vi "CRYGraph Property Window Table.vi"(8 "Tab Name":string, 9 "Graph VI Ref":refnum<vi>) -> ()   [LabVIEW 2013]
uses:
  Control/CRYTable Property.ctl
panel:
  in  "Redraw":bool
  in  "Draw":bool
  in  "Table Property":T1 {"Precision" items=["Digits of precision", "Significant digits"]}
  in  "OK":bool
  in  "List Tab":enum32{"Title", "Format"}(tab) caption="Table Tab"
  in  "Title Name":string caption="标题名字"
  in  "Show vertical scroll bar":bool caption="显示垂直滚动条"
  in  "Show horizontal scroll bar":bool caption="显示水平滚动条"
  in  "Row Header Width":u16
  in  "Column Width":u16
  in  "Hide Traling Zeros":bool caption="隐藏尾随零"
  in  "PrecisionType":u16(ring) caption="Precision" items=["精度位数", "有效数字"]
  in  "Digits":u16
  in  "Notation":u16(slide)
  in  "Display Units":bool caption="显示单位"
  in  "Transpose":bool
  in  "Reset All Columns":bool
  out "Number Format":bool caption="数字格式"
  out "Options":bool caption="表选项"
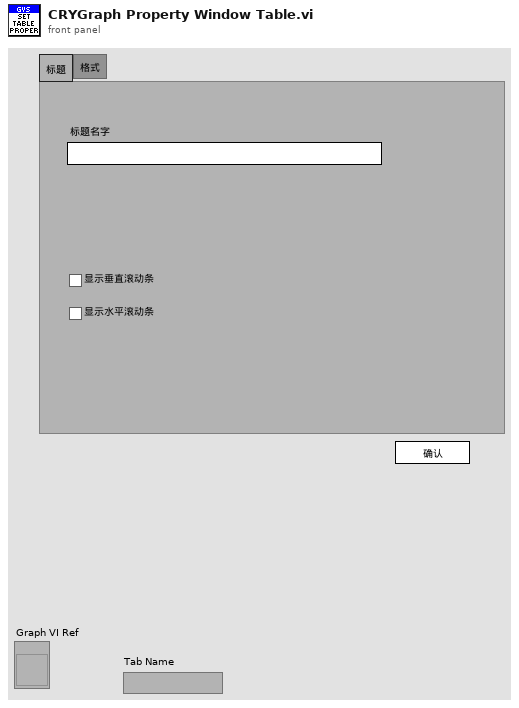
[diagram p1: front panel]
types:
  T1 = typedef "CRYTable Property.ctl" = cluster{"Reset All Columns":bool, "Transpose":bool, "Display Units":bool, "Notation":u16, "Digits":u16, "Precision":u16, "Hide Traling Zeros":bool, "Column Width":u16, "Row Header Width":u16, "Show vertical scroll bar":bool, "Show horizontal scroll bar":bool}
  T2 = enum32{"Page Enabled", "Page Disabled", "Page Disabled & Grayed"}
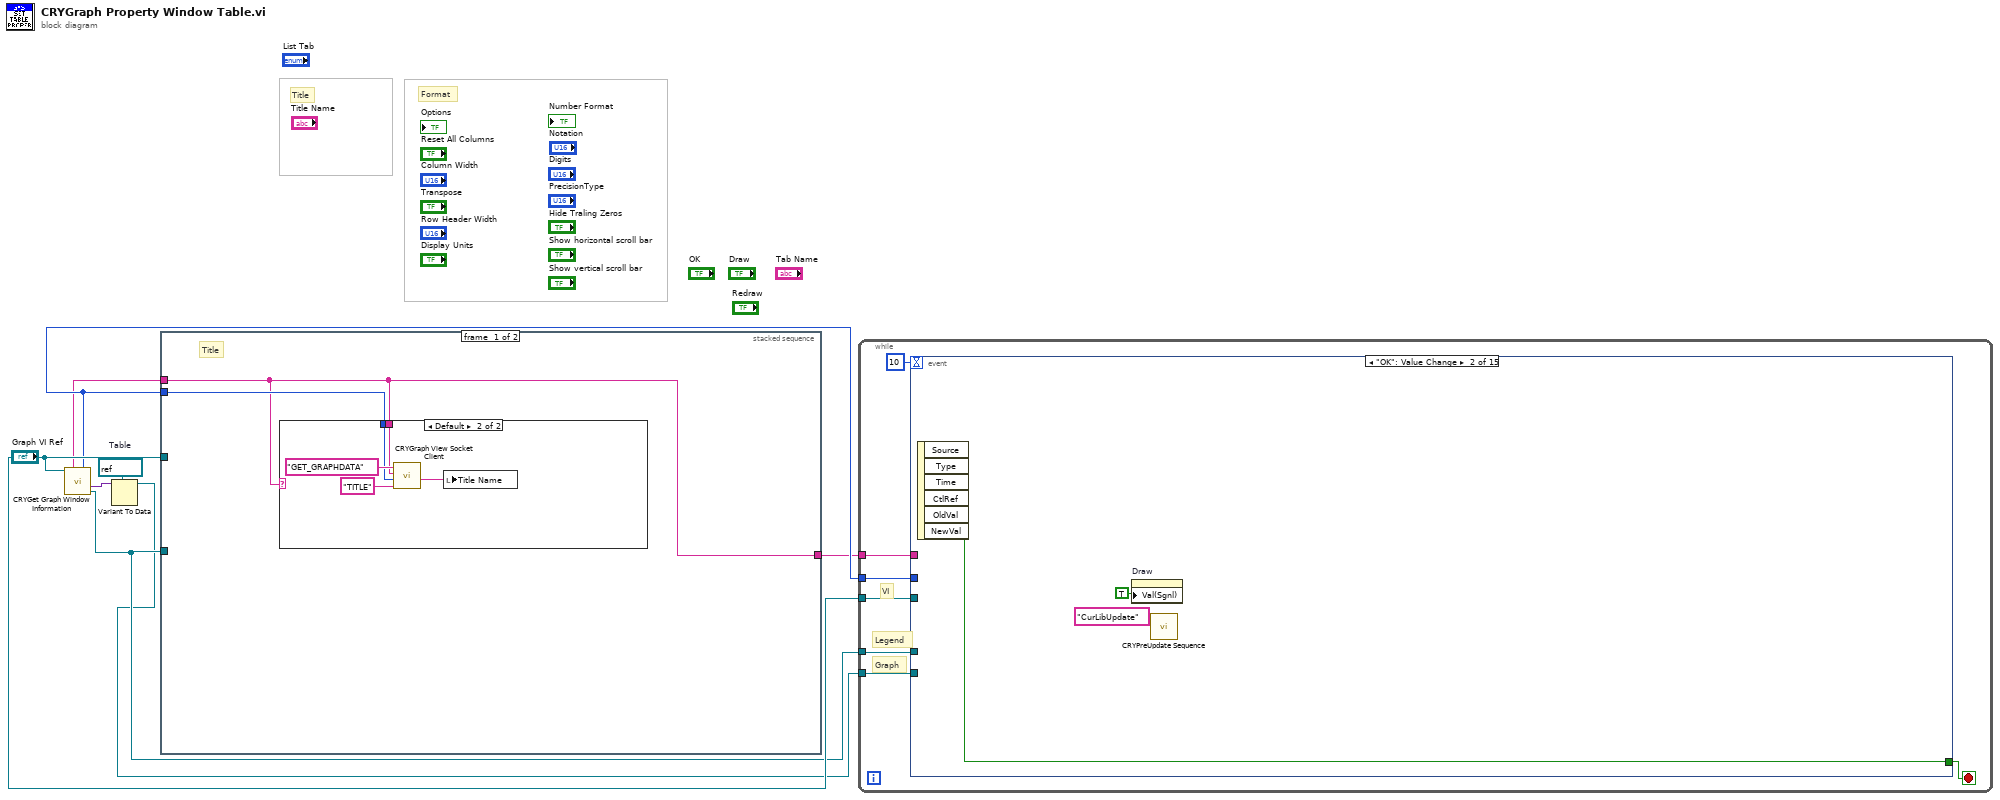
[diagram p0: block diagram]
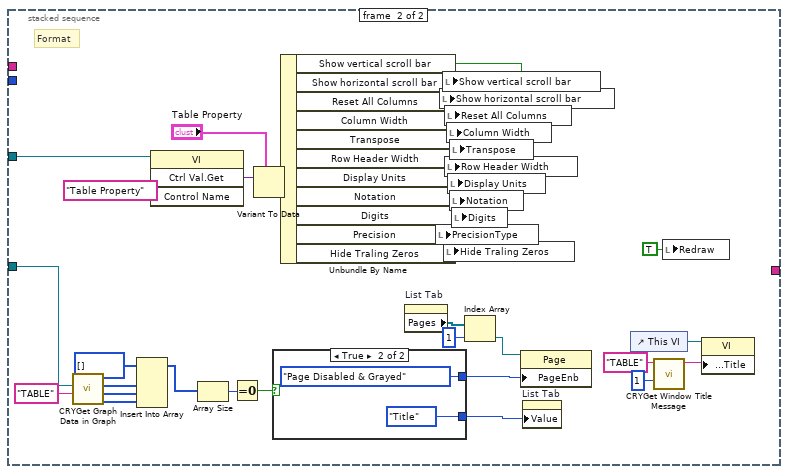
[diagram p3: hidden frame]
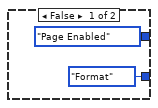
[diagram p4: hidden frame]
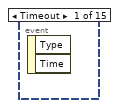
[diagram p5: hidden frame]
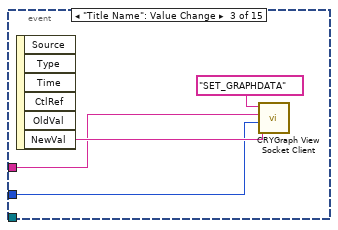
[diagram p6: hidden frame]
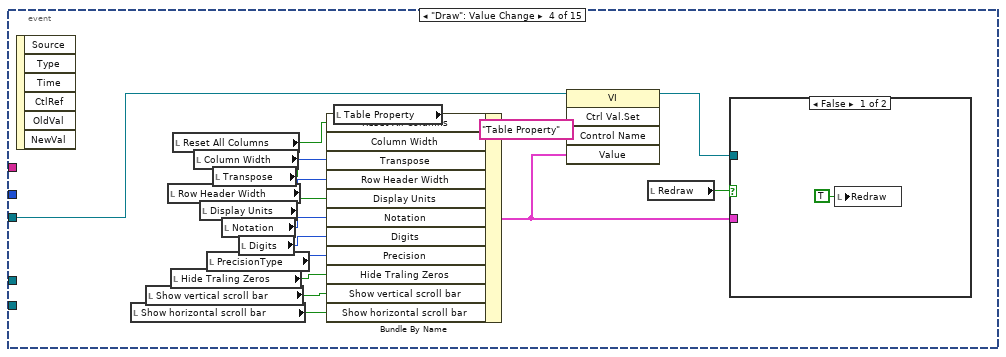
[diagram p7: hidden frame]
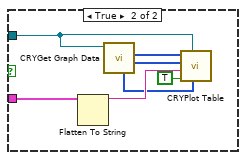
[diagram p8: hidden frame]
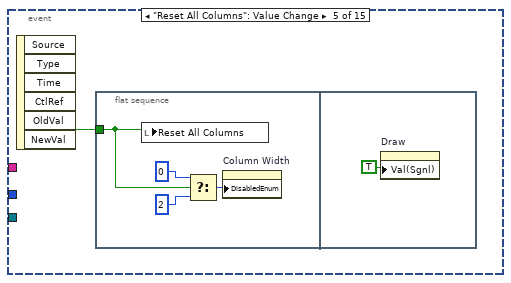
[diagram p9: hidden frame]
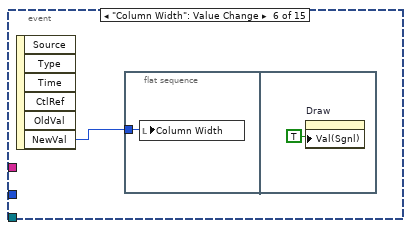
[diagram p10: hidden frame]
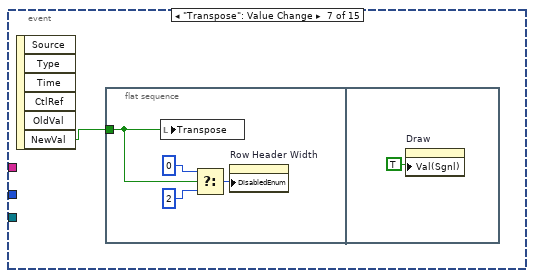
[diagram p11: hidden frame]
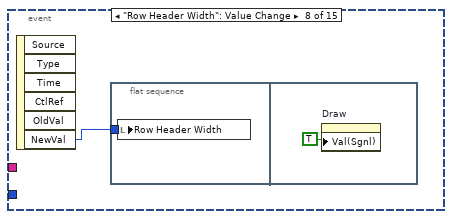
[diagram p12: hidden frame]
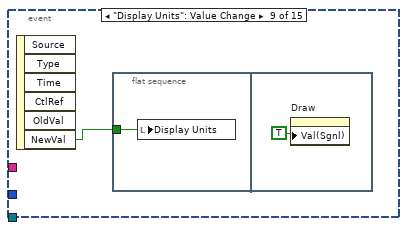
[diagram p13: hidden frame]
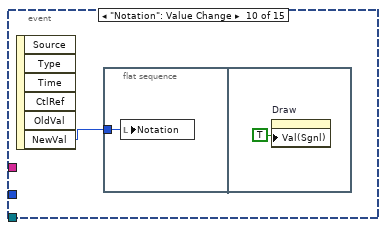
[diagram p14: hidden frame]
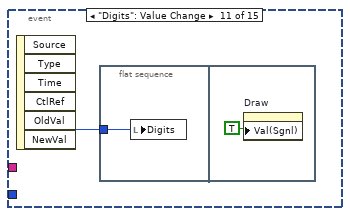
[diagram p15: hidden frame]
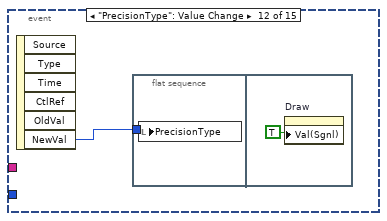
[diagram p16: hidden frame]
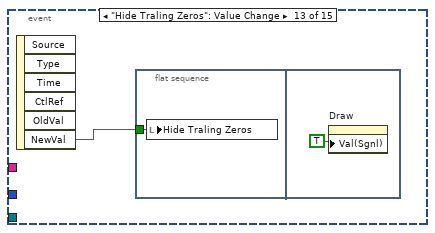
[diagram p17: hidden frame]
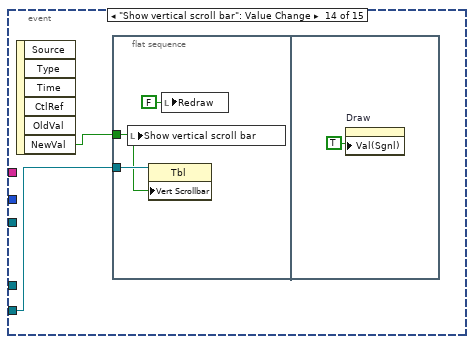
[diagram p18: hidden frame]
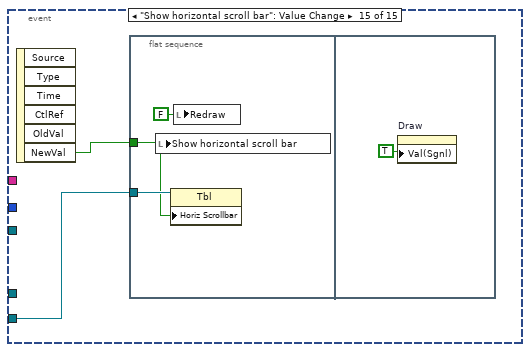
[diagram p19: hidden frame]
diagram:
  w1 = refnum<vi> refnum  # Table
  # "Title"
  # "Format"
  n1 = call "CRYGet Graph Window Information.vi"("pGraph VI In"="Graph VI Ref") -> ("Queue Name Out"=w6:string, "Graph Number Out"=w7:i32, "Graph Control Ref Out"=w2:variant, "Legend Ref Out"=w4:refnum<vi>)  [unwired: 2 in, 9 out]
  n2 = Variant To Data(type=w1, Variant=w2) -> (data=w3:refnum<vi>)  [unwired: 1 in, 1 out]
  n3 = stacked-sequence {
    tunnel: "Graph VI Ref" -> [_ w48]
    tunnel: w4 -> [_ w23]
    tunnel: w7 -> [w10 _]
    tunnel: w6 -> [w9 _]
    tunnel: [w9 _] -> w5
    frame #0 {
      # "Title"
      n4 = case shown="Default" w9 {
        tunnel: w10 -> [_ w13]
        tunnel: w9 -> [_ w12]
        frame "test DataView" {
        }
        frame Default {
          n5 = call "CRYGraph View Socket Client.vi"("sOption"="TITLE", "nData"=w13, "sData"=w12, "sAction"="GET_GRAPHDATA") -> ("sData Out"=w11:string)  [unwired: 4 in, 3 out]
          n6 = local write "Title Name"(w11) -> ()
        }
      }
    }
    frame #1 {
      # "Format"
      n7 = call "CRYGet Graph Data in Graph.vi"("Graph Type"="TABLE", "Legend Refnum"=w23) -> ("Result Rows"=w26:i32[], "Value Rows"=w27:i32[], "Rows"=w28:i32[])  [unwired: 2 in, 5 out]
      n8 = Insert Into Array(array=i32[] [], new element #1=w28, new element #2=w27, new element #3=w26) -> (w24:i32[])  [unwired: 1 in]
      n9 = invoke class="VI" method="Ctrl Val.Get"(reference=w48, "Control Name"="Table Property") -> ("Get Control Value Variant"=w49:variant)  [unwired: 2 in, 3 out]
      n10 = Array Size(array=w24) -> (size(s)=w36:i32)
      n11 = Equal To 0?(x=w36) -> (x = 0?=w33:bool)
      n12 = Variant To Data(type="Table Property", Variant=w49) -> (data=w46:T1)  [unwired: 1 in, 1 out]
      n13 = case shown="True" w33 {
        tunnel: [T2."Page Enabled" ("Page Enabled State") T2."Page Disabled & Grayed" ("Page Enabled State")] -> w31
        tunnel: [enum32{"Title", "Format"}."Format" ("Tab Control") enum32{"Title", "Format"}."Title" ("Tab Control")] -> w30
        frame False {
        }
        frame True {
        }
      }
      n14 = Unbundle By Name(w46) -> ("Show vertical scroll bar"=w18:bool, "Show horizontal scroll bar"=w17:bool, "Reset All Columns"=w45:bool, "Column Width"=w44:u16, "Transpose"=w43:bool, "Row Header Width"=w42:u16, "Display Units"=w41:bool, "Notation"=w40:u16, "Digits"=w39:u16, "Precision"=w38:u16, "Hide Traling Zeros"=w37:bool)
      n15 = property on="List Tab" class="TabCtl (strict)"() -> ("Pages"=w35:refnum<vi>[])  [unwired: 2 in, 2 out]
      n16 = local write "PrecisionType"(w38) -> ()
      n17 = local write "Show horizontal scroll bar"(w17) -> ()
      n18 = local write "Show vertical scroll bar"(w18) -> ()
      n19 = local write "Hide Traling Zeros"(w37) -> ()
      n20 = local write "Reset All Columns"(w45) -> ()
      n21 = local write "Row Header Width"(w42) -> ()
      n22 = local write "Column Width"(w44) -> ()
      n23 = local write "Display Units"(w41) -> ()
      n24 = local write "Transpose"(w43) -> ()
      n25 = local write "Notation"(w40) -> ()
      n26 = local write "Digits"(w39) -> ()
      n27 = Index Array(array=w35, index=1) -> (element=w32:refnum<vi>)
      n28 = property class="Page"(reference=w32, "PageEnb"=w31) -> ()  [unwired: 1 in, 2 out]
      n29 = property on="List Tab" class="TabCtl (strict)"("Value"=w30) -> ()  [unwired: 2 in, 2 out]
      n30 = control-ref of="This VI"() -> (w19:refnum<vi>)
      n31 = call "CRYGet Window Title Message.vi"("No"=1 ("Error No"), "Kind"="TABLE") -> ("Multibyte String"=w20:string)  [unwired: 4 in, 5 out]
      n32 = local write "Redraw"(TRUE ("Redraw")) -> ()
      n33 = property class="VI"(reference=w19, "Front Panel.Title"=w20) -> ()  [unwired: 1 in, 2 out]
    }
  }
  n34 = while {
    tunnel: w7 -> [w60]
    tunnel: "Graph VI Ref" -> [w59]
    tunnel: w4 -> [w58]
    tunnel: w5 -> [w56]
    tunnel: w3 -> [w55]
    stop <- w57 stop-if-true
    # "Graph"
    # "Legend"
    # "VI"
    n35 = event shown="[1] \"OK\": Value Change" {
      selector: _ -> [_ _ _ _ _ _ _ _ _ _ _ _ _ _ _]
      dyn-events: _ -> [_ _ _ _ _ _ _ _ _ _ _ _ _ _ _]
      timeout: 10 -> [_ _ _ _ _ _ _ _ _ _ _ _ _ _ _]
      tunnel: [_ w64 _ _ _ _ _ _ _ _ _ _ _ _ _] -> w57
      tunnel: w60 -> [_ _ w65 _ _ _ _ _ _ _ _ _ _ _ _]
      tunnel: w59 -> [_ _ _ w83 _ _ _ _ _ _ _ _ _ _ _]
      tunnel: w58 -> [_ _ _ _ _ _ _ _ _ _ _ _ _ _ _]
      tunnel: w56 -> [_ _ w66 _ _ _ _ _ _ _ _ _ _ _ _]
      tunnel: w55 -> [_ _ _ _ _ _ _ _ _ _ _ _ _ w128 w134]
      event Timeout {
        n36 = event-data() -> ()  [unwired: 3 out]
      }
      event "OK": Value Change {
        n37 = event-data() -> ("NewVal"=w64:bool)  [unwired: 6 out]
        n38 = property on="Draw" class="Bool (strict)"("Val(Sgnl)"=TRUE ("Value (Signaling)")) -> ()  [unwired: 2 in, 2 out]
        n39 = call "CRYPreUpdate Sequence.vi"("EventName"="CurLibUpdate") -> ()  [unwired: 15 in]
      }
      event "Title Name": Value Change {
        n40 = event-data() -> ("NewVal"=w67:string)  [unwired: 6 out]
        n41 = call "CRYGraph View Socket Client.vi"("sOption"=w67, "nData"=w65, "sData"=w66, "sAction"="SET_GRAPHDATA") -> ()  [unwired: 4 in, 4 out]
      }
      event "Draw": Value Change {
        n42 = event-data() -> ()  [unwired: 7 out]
        n43 = local read "Show horizontal scroll bar"() -> (w70:bool)
        n44 = local read "Show vertical scroll bar"() -> (w71:bool)
        n45 = local read "Row Header Width"() -> (w77:u16)
        n46 = local read "Hide Traling Zeros"() -> (w72:bool)
        n47 = local read "Reset All Columns"() -> (w80:bool)
        n48 = local read "Column Width"() -> (w79:u16)
        n49 = local read "Display Units"() -> (w76:bool)
        n50 = local read "PrecisionType"() -> (w73:u16)
        n51 = local read "Transpose"() -> (w78:bool)
        n52 = local read "Notation"() -> (w75:u16)
        n53 = local read "Digits"() -> (w74:u16)
        n54 = local read "Table Property"() -> (w81:T1)
        n55 = Bundle By Name(cluster=w81, "Reset All Columns"=w80, "Column Width"=w79, "Transpose"=w78, "Row Header Width"=w77, "Display Units"=w76, "Notation"=w75, "Digits"=w74, "Precision"=w73, "Hide Traling Zeros"=w72, "Show vertical scroll bar"=w71, "Show horizontal scroll bar"=w70) -> (w84:T1)
        n56 = invoke class="VI" method="Ctrl Val.Set"(reference=w83, "Control Name"="Table Property", "Value"=w84) -> (reference out=w85:refnum<vi>)  [unwired: 2 in, 4 out]
        n57 = local read "Redraw"() -> (w69:bool)
        n58 = case shown="False" w69 {
          tunnel: w84 -> [_ w91]
          tunnel: w85 -> [_ w87]
          frame False {
            n59 = local write "Redraw"(TRUE ("Redraw")) -> ()
          }
          frame True {
            n60 = Flatten To String(anything=w91) -> (data string=w90:string)  [unwired: 3 in, 2 out]
            n61 = call "CRYGet Graph Data.vi"("pGraph VI"=w87) -> ("Value Rows"=w92:i32[], "Rows"=w93:i32[], "Result Rows"=w88:i32[])  [unwired: 2 in, 6 out]
            n62 = call "CRYPlot Table.vi"("Result Rows In"=w88, "pGraph VI In"=w87, "Graph Set?"=TRUE, "Flattened Property"=w90, "Value Rows In"=w92, "Curve Rows In"=w93) -> ()  [unwired: 6 out]
          }
        }
      }
      event "Reset All Columns": Value Change {
        n63 = event-data() -> ("NewVal"=w94:bool)  [unwired: 6 out]
        n64 = flat-sequence {
          tunnel: w94 -> [w96]
          frame #0 {
            n65 = local write "Reset All Columns"(w96) -> ()
            n66 = Select(t=u16 0 ("Column Width"), s=w96, f=u16 2 ("Column Width")) -> (s? t:f=w95:u16)
            n67 = property on="Column Width" class="DigNum (strict)"("DisabledEnum"=w95) -> ()  [unwired: 2 in, 2 out]
          }
          frame #1 {
            n68 = property on="Draw" class="Bool (strict)"("Val(Sgnl)"=TRUE ("Value (Signaling)")) -> ()  [unwired: 2 in, 2 out]
          }
        }
      }
      event "Column Width": Value Change {
        n69 = event-data() -> ("NewVal"=w100:u16)  [unwired: 6 out]
        n70 = flat-sequence {
          tunnel: w100 -> [w101]
          frame #0 {
            n71 = local write "Column Width"(w101) -> ()
          }
          frame #1 {
            n72 = property on="Draw" class="Bool (strict)"("Val(Sgnl)"=TRUE ("Value (Signaling)")) -> ()  [unwired: 2 in, 2 out]
          }
        }
      }
      event "Transpose": Value Change {
        n73 = event-data() -> ("NewVal"=w103:bool)  [unwired: 6 out]
        n74 = flat-sequence {
          tunnel: w103 -> [w104]
          frame #0 {
            n75 = local write "Transpose"(w104) -> ()
            n76 = Select(t=u16 0 ("Column Width"), s=w104, f=u16 2 ("Column Width")) -> (s? t:f=w105:u16)
            n77 = property on="Row Header Width" class="DigNum (strict)"("DisabledEnum"=w105) -> ()  [unwired: 2 in, 2 out]
          }
          frame #1 {
            n78 = property on="Draw" class="Bool (strict)"("Val(Sgnl)"=TRUE ("Value (Signaling)")) -> ()  [unwired: 2 in, 2 out]
          }
        }
      }
      event "Row Header Width": Value Change {
        n79 = event-data() -> ("NewVal"=w109:u16)  [unwired: 6 out]
        n80 = flat-sequence {
          tunnel: w109 -> [w110]
          frame #0 {
            n81 = local write "Row Header Width"(w110) -> ()
          }
          frame #1 {
            n82 = property on="Draw" class="Bool (strict)"("Val(Sgnl)"=TRUE ("Value (Signaling)")) -> ()  [unwired: 2 in, 2 out]
          }
        }
      }
      event "Display Units": Value Change {
        n83 = event-data() -> ("NewVal"=w112:bool)  [unwired: 6 out]
        n84 = flat-sequence {
          tunnel: w112 -> [w113]
          frame #0 {
            n85 = local write "Display Units"(w113) -> ()
          }
          frame #1 {
            n86 = property on="Draw" class="Bool (strict)"("Val(Sgnl)"=TRUE ("Value (Signaling)")) -> ()  [unwired: 2 in, 2 out]
          }
        }
      }
      event "Notation": Value Change {
        n87 = event-data() -> ("NewVal"=w115:u16)  [unwired: 6 out]
        n88 = flat-sequence {
          tunnel: w115 -> [w116]
          frame #0 {
            n89 = local write "Notation"(w116) -> ()
          }
          frame #1 {
            n90 = property on="Draw" class="Bool (strict)"("Val(Sgnl)"=TRUE ("Value (Signaling)")) -> ()  [unwired: 2 in, 2 out]
          }
        }
      }
      event "Digits": Value Change {
        n91 = event-data() -> ("NewVal"=w118:u16)  [unwired: 6 out]
        n92 = flat-sequence {
          tunnel: w118 -> [w119]
          frame #0 {
            n93 = local write "Digits"(w119) -> ()
          }
          frame #1 {
            n94 = property on="Draw" class="Bool (strict)"("Val(Sgnl)"=TRUE ("Value (Signaling)")) -> ()  [unwired: 2 in, 2 out]
          }
        }
      }
      event "PrecisionType": Value Change {
        n95 = event-data() -> ("NewVal"=w121:u16)  [unwired: 6 out]
        n96 = flat-sequence {
          tunnel: w121 -> [w122]
          frame #0 {
            n97 = local write "PrecisionType"(w122) -> ()
          }
          frame #1 {
            n98 = property on="Draw" class="Bool (strict)"("Val(Sgnl)"=TRUE ("Value (Signaling)")) -> ()  [unwired: 2 in, 2 out]
          }
        }
      }
      event "Hide Traling Zeros": Value Change {
        n99 = event-data() -> ("NewVal"=w124:bool)  [unwired: 6 out]
        n100 = flat-sequence {
          tunnel: w124 -> [w125]
          frame #0 {
            n101 = local write "Hide Traling Zeros"(w125) -> ()
          }
          frame #1 {
            n102 = property on="Draw" class="Bool (strict)"("Val(Sgnl)"=TRUE ("Value (Signaling)")) -> ()  [unwired: 2 in, 2 out]
          }
        }
      }
      event "Show vertical scroll bar": Value Change {
        n103 = event-data() -> ("NewVal"=w127:bool)  [unwired: 6 out]
        n104 = flat-sequence {
          tunnel: w128 -> [w130]
          tunnel: w127 -> [w129]
          frame #0 {
            n105 = local write "Show vertical scroll bar"(w129) -> ()
            n106 = property class="Tbl"(reference=w130, "Vert Scrollbar"=w129) -> ()  [unwired: 1 in, 2 out]
            n107 = local write "Redraw"(FALSE ("Redraw")) -> ()
          }
          frame #1 {
            n108 = property on="Draw" class="Bool (strict)"("Val(Sgnl)"=TRUE ("Value (Signaling)")) -> ()  [unwired: 2 in, 2 out]
          }
        }
      }
      event "Show horizontal scroll bar": Value Change {
        n109 = event-data() -> ("NewVal"=w133:bool)  [unwired: 6 out]
        n110 = flat-sequence {
          tunnel: w134 -> [w136]
          tunnel: w133 -> [w135]
          frame #0 {
            n111 = local write "Show horizontal scroll bar"(w135) -> ()
            n112 = property class="Tbl"(reference=w136, "Horiz Scrollbar"=w135) -> ()  [unwired: 1 in, 2 out]
            n113 = local write "Redraw"(FALSE ("Redraw")) -> ()
          }
          frame #1 {
            n114 = property on="Draw" class="Bool (strict)"("Val(Sgnl)"=TRUE ("Value (Signaling)")) -> ()  [unwired: 2 in, 2 out]
          }
        }
      }
    }
  }
